vi "pp2_updateDAQOutput.vi"() -> ()   [LabVIEW 2013]
uses:
  pp2_State.ctl
  pp2_CTL_StateInfo.ctl
  pp2_TrialType.ctl
  labolabo2/waveforms/WFTypes.ctl
  pp2_Trial.ctl
panel:
  in  "Side Changed?":bool
  in  "State Changed?":bool
  out "DAQ Out":T1
  in  "DAQ In":T2
  in  "State In":T3={"Curr  tr"=0, "Curr (ms)"=0, "Cum (ms)"=0, "Run loop diff"=0, "Exit (ms)"=0, "Curr State"=enum."0 Initialization", "Prev State"=enum."0 Initialization", "Side"=FALSE, "Sw1"=FALSE, "Tone Gate"=FALSE, "Stim"=FALSE, "Sw2"=FALSE, "Curr code"=0, "Current Trial"={"Trial Type Number"=1, "Trial Type"=enum."GO", "Trial Weight"=100, "Shock (mA)"=0.3, "Duration (ms)"=0.25, "Type"=enum."04 FM Sweep", "Stim P2"=4000.0, "Stim P3"=0.0, "Stim P4"=0.0, "Stim P1"=2000.0}, "Last tone"=0, "Countdown (s)"=0} {"Current Trial"."Shock (mA)" min=-1.0 max=5.0; "Current Trial"."Trial Weight" step=1; "Current Trial"."Duration (ms)" min=0.0 max=1.0; "Current Trial"."Trial Type Number" min=1 max=256 step=1; "Curr code" format="%b"}
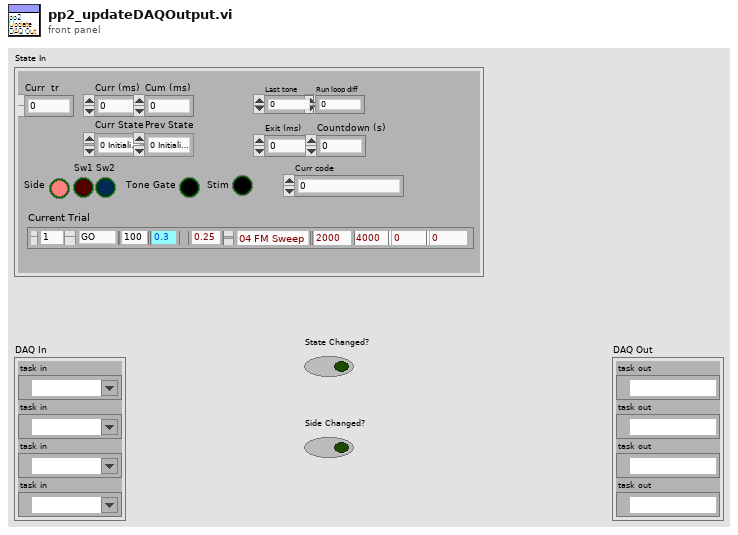
[diagram p1: front panel]
types:
  T1 = cluster{"task out":refnum<k21>, "task out":refnum<k21>, "task out":refnum<k21>, "task out":refnum<k21>}
  T2 = cluster{"task in":refnum<k21>, "task in":refnum<k21>, "task in":refnum<k21>, "task in":refnum<k21>}
  T3 = typedef "pp2_CTL_StateInfo.ctl" = cluster{"Curr  tr":u16, "Curr (ms)":i64, "Cum (ms)":i64, "Run loop diff":i64, "Exit (ms)":i64, "Curr State":T4, "Prev State":T4, "Side":bool, "Sw1":bool, "Tone Gate":bool, "Stim":bool, "Sw2":bool, "Curr code":u8, "Current Trial":T5, "Last tone":i64, "Countdown (s)":i64}
  T4 = typedef "pp2_State.ctl" = enum8{"0 Initialization", "1 Habituation", "2 Load next", "3 Wait", "4 GO Trial", "5 GO Jumped", "6 GO Timeout", "7 NOGO Trial", "8 NOGO Jumped", "9 NOGO Timeout", "10 TEST Trial", "11 TEST Jumped", "12 TEST Timeout", "13 Done"}
  T5 = typedef "pp2_Trial.ctl" = cluster{"Trial Type Number":i16, "Trial Type":T6, "Trial Weight":u32, "Shock (mA)":dbl, "Duration (ms)":dbl, "Type":T7, "Stim P2":dbl, "Stim P3":dbl, "Stim P4":dbl, "Stim P1":dbl}
  T6 = typedef "pp2_TrialType.ctl" = enum16{"OFF", "GO", "NOGO", "TEST"}
  T7 = typedef "WFTypes.ctl" = enum16{"00 NULL", "01 DC", "02 Noise", "03 Pure Tone", "04 FM Sweep"}
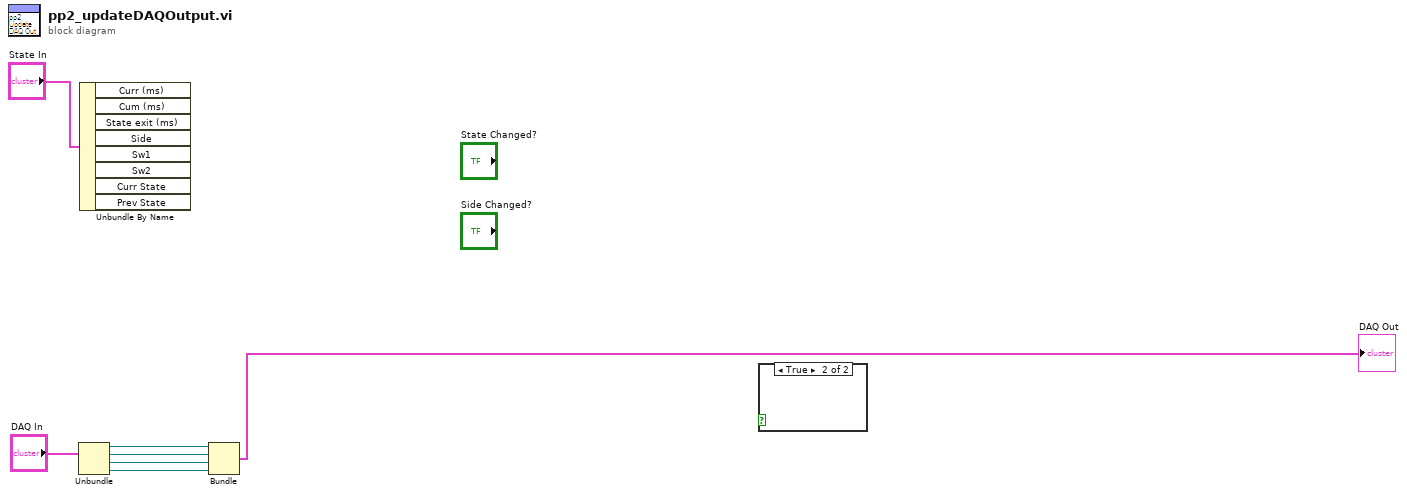
[diagram p0: block diagram]
diagram:
  n1 = Unbundle("DAQ In") -> ("task in"=w5:refnum<k21>, "task in"=w4:refnum<k21>, "task in"=w3:refnum<k21>, "task in"=w1:refnum<k21>)
  n2 = Unbundle By Name("State In") -> ()  [unwired: 8 out]
  n3 = Bundle("task in"=w5, "task in"=w4, "task in"=w3, "task in"=w1) -> (→"DAQ Out":T2)  [unwired: 1 in]
  n4 = case shown="True" {
    selector: _ -> [_ _]
    frame False {
    }
    frame True {
    }
  }
